vi "Gradient  BG Color.vi"(6 "Row or Col Option":T1, 8 "错误输入":errorcluster, 9 "Second BG Color":u32(colorbox)=9868950, 10 "First BG Color":u32(colorbox)=16448250, 11 "Table Ref In":refnum<vi>) -> (0 "错误输出":errorcluster, 3 "Table Ref Out":refnum<vi>)   [LabVIEW 2012, in "Table Tool.lvlib"]
uses:
  Table Tool.lvlib
  Custum Type/Selet Row or Col.ctl
  Custum Type/GetOrSet.ctl
  Property/Set Or Get Num of Rows or Cols.vi
  Property/Set Or get ActiveCell Bk Color.vi
  Property/Set  ActiveCell by Row Or Column.vi
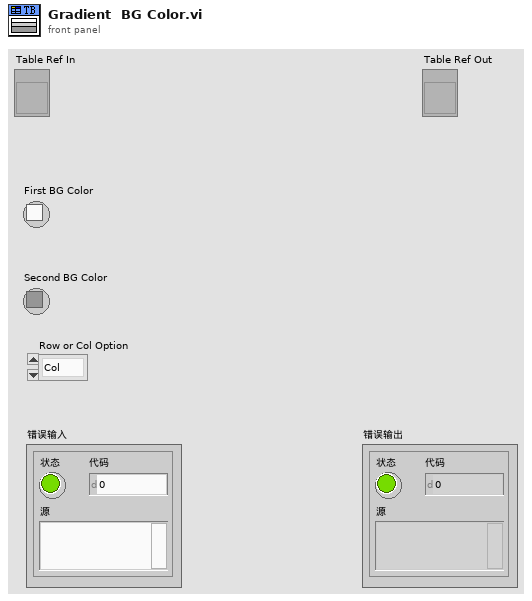
[diagram p1: front panel]
types:
  T1 = typedef "Table Tool.lvlib/Selet Row or Col.ctl" = enum16{"Col", "Row"}
  T2 = typedef "Table Tool.lvlib/GetOrSet.ctl" = enum16{"Get", "Set"}
  T3 = enum16{"All Rows and Cols", "Row Head", "Col Head", "N Row", "N Col"}
  T4 = typedef "LVRowAndColumnTypeDef.ctl" = cluster{"Row":i32, "Column":i32}
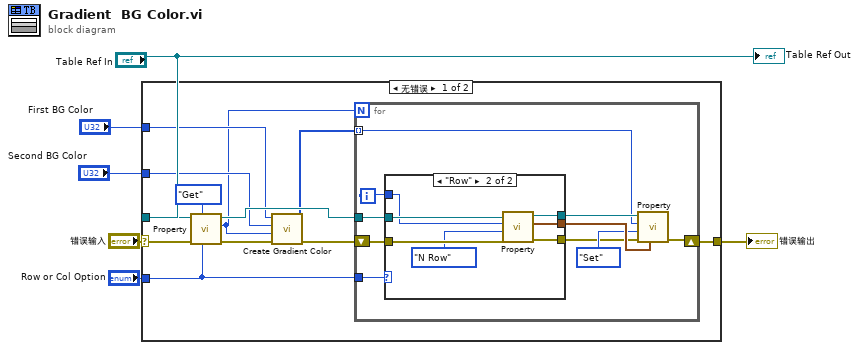
[diagram p0: block diagram]
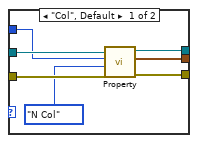
[diagram p2: hidden frame]
diagram:
  n1 = case shown="无错误" "错误输入" {
    selector: "错误输入" -> [w18 w43]
    tunnel: [w13 w43] -> w5
    tunnel: "Row or Col Option" -> [w15 _]
    tunnel: "Table Ref In" -> [w17 _]
    tunnel: "First BG Color" -> [w10 _]
    tunnel: "Second BG Color" -> [w9 _]
    frame No Error {
      n2 = call-poly "Property.vi"("Row or Col Option"=w15, "Mode"=GetOrSet."Get", "error in (no error)"=w18, "Table Ref In"=w17) -> ("error out"=w12:errorcluster, "Number of Rows or Cols Out"=w7:u32, "Table Ref Out"=w14:refnum<vi>)  [unwired: 5 in]
      n3 = call "Create Gradient Color.vi"("错误输入"=w12, "Length"=w7, "End"=w9, "Start"=w10) -> ("错误输出"=w11:errorcluster, "ColorArray"=w8:u32[])  [unwired: 6 in]
      n4 = for {
        N: w7 -> [_]
        tunnel: w15 -> [w25]
        tunnel: w14 -> [w28]
        shift-right: [w21] -> w13
        shift-left: w11 -> [w26]
        tunnel: w8 -> [w19] mode=indexing
        i -> [w23]
        n5 = case shown="\"Row\"" w25 {
          tunnel: w28 -> [w32 w42]
          tunnel: [w35 w41] -> w27
          tunnel: w26 -> [w31 w40]
          tunnel: [w34 w39] -> w20
          tunnel: w23 -> [w30 w37]
          tunnel: [w33 w36] -> w24
          frame "Col", Default {
            n6 = call-poly "Property.vi"("error in (no error)"=w31, "Option"=T3."N Col", "N"=w30, "Table Ref In"=w32) -> ("error out"=w34:errorcluster, "ActiveCell Out"=w33:T4, "Table Ref Out"=w35:refnum<vi>)  [unwired: 5 in]
          }
          frame "Row" {
            n7 = call-poly "Property.vi"("error in (no error)"=w40, "Option"=T3."N Row", "N"=w37, "Table Ref In"=w42) -> ("error out"=w39:errorcluster, "ActiveCell Out"=w36:T4, "Table Ref Out"=w41:refnum<vi>)  [unwired: 5 in]
          }
        }
        n8 = call-poly "Property.vi"("Active Cell"=w24, "error in (no error)"=w20, "Mode"=GetOrSet."Set", "BK Color In"=w19, "Table Ref In"=w27) -> ("error out"=w21:errorcluster)  [unwired: 4 in, 2 out]
      }
    }
    frame Error {
    }
  }
  "错误输出" <- w5
  "Table Ref Out" <- "Table Ref In"
